vi "AB_1200_1100_Project_DestinationItems.vi"(6 "usedDestinations":i32[](array[numeric]), 7 "action":T2, 8 "error in (no error)":errorcluster, 9 "buildTypeGUID":string, 10 "oldBuildObject":T1, 11 "buildObject":T1) -> (0 "error out":errorcluster, 3 "buildObject out":T1)   [LabVIEW 2020]
doc: "Reads and writes the data to the object property bag."
uses:
  <resource>/Framework/Providers/API/ItemRef.ctl
  <vilib>/AppBuilder/RW_Project/AB_RW_Project_PropBag_ArrayAction.ctl
  <vilib>/AppBuilder/RW_Project/AB_RW_Project_PropBag_Action.ctl
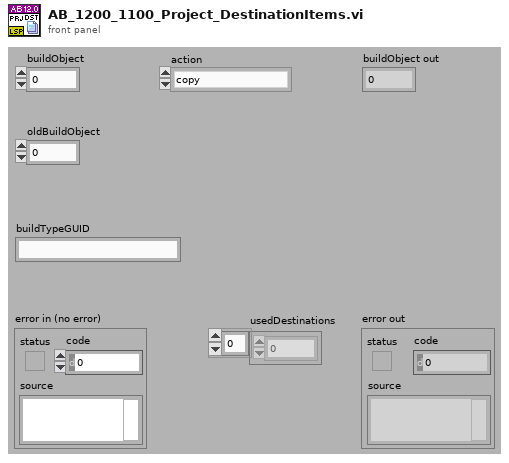
[diagram p1: front panel]
types:
  T1 = typedef "ItemRef.ctl" = u64
  T2 = typedef "AB_RW_Project_PropBag_ArrayAction.ctl" = enum16{"copy", "saveForPrevious", "loadFromPrevious", "clear"}
  T3 = typedef "AB_RW_Project_PropBag_Action.ctl" = enum16{"read", "write", "clear", "readPrevious", "writePrevious", "clearPrevious"}
  T4 = cluster{"destName":string, "path":path, "preserveHierarchy":bool, "libraryName":string}
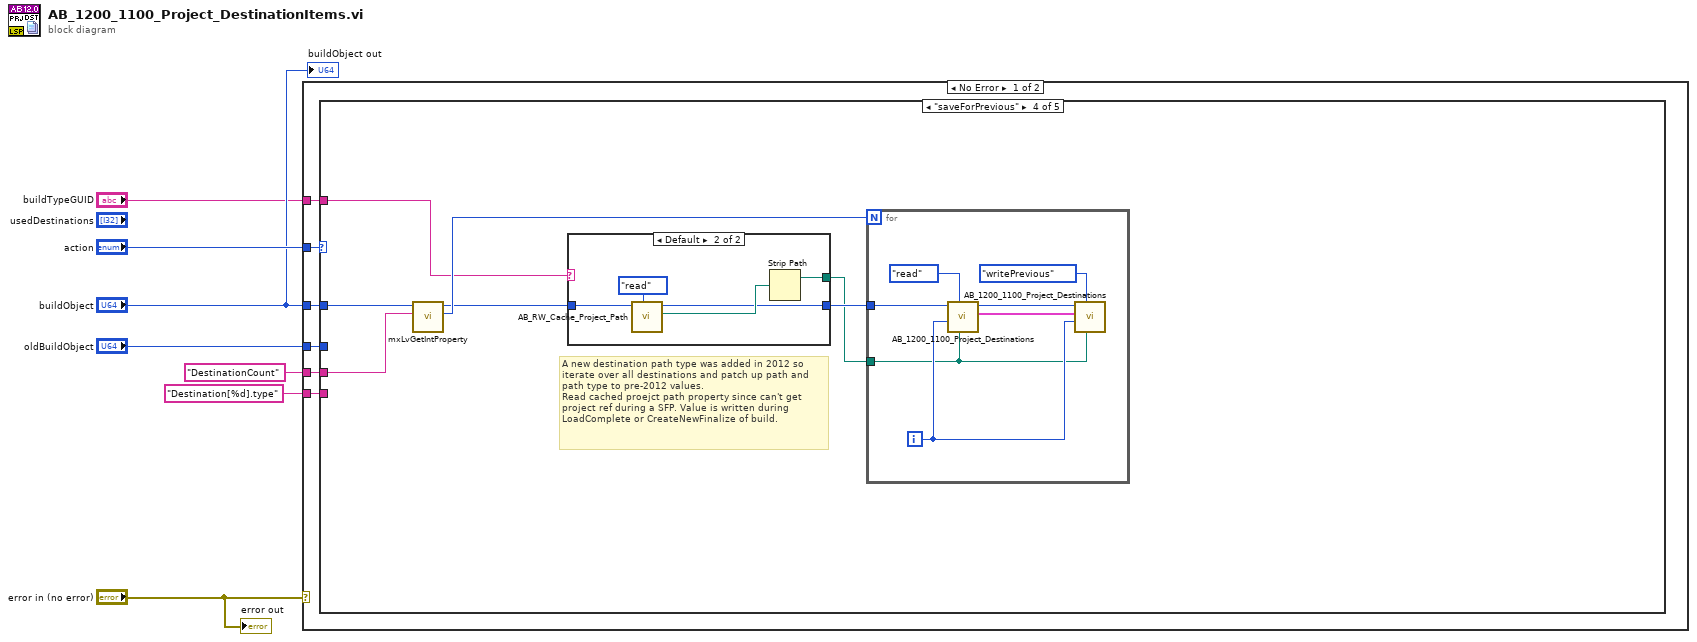
[diagram p0: block diagram]
diagram:
  n1 = case shown="No Error" "error in (no error)" {
    tunnel: "action" -> [w13 _]
    tunnel: "buildObject" -> [w12 _]
    tunnel: "DestinationCount" -> [w11 _]
    tunnel: "Destination[%d].type" -> [w10 _]
    tunnel: "oldBuildObject" -> [w9 _]
    tunnel: "buildTypeGUID" -> [w8 _]
    frame No Error {
      n2 = case shown="\"saveForPrevious\"" w13 {
        tunnel: w12 -> [_ _ _ w19 _]
        tunnel: w11 -> [_ _ _ w18 _]
        tunnel: w10 -> [_ _ _ _ _]
        tunnel: w9 -> [_ _ _ _ _]
        tunnel: w8 -> [_ _ _ w15 _]
        frame Default {
        }
        frame "loadFromPrevious" {
        }
        frame "copy" {
        }
        frame "saveForPrevious" {
          # "A new destination path type was added in 2012 so iterate over all destinations and patch up path and path type to pre-2012 values. \nRead cached proejct path property since can't get project ref during a SFP. Value is written during LoadComplete or CreateNewFinalize of build."
          n3 = call <resource>:"mxLvGetIntProperty.vi"("Tag"=w18, "Item"=w19) -> ("Value"=w20:i32, "Item"=w17:T1)  [unwired: 7 in, 1 out]
          n4 = case shown="Default" w15 {
            tunnel: w17 -> [w21 w23]
            tunnel: [w21 w22] -> w16
            tunnel: [_ w26] -> w14
            frame "{69A947D5-514E-4E75-818E-69657C0547D8}" {
              # "For RTEXE, destination items are saved as absolute"
            }
            frame Default {
              n5 = call <vilib>:"AB_RW_Cache_Project_Path.vi"("action"=AB_RW_Project_PropBag_Action."read", "buildObject"=w23) -> ("ProjectPath out"=w24:path, "buildObject out"=w22:T1)  [unwired: 7 in, 1 out]
              n6 = Strip Path(path=w24) -> (stripped path=w26:path)  [unwired: 1 out]
            }
          }
          n7 = for {
            N: w20 -> [_]
            tunnel: w16 -> [w32]
            tunnel: w14 -> [w28]
            i -> [w29]
            n8 = call <vilib>:"AB_1200_1100_Project_Destinations.vi"("ProjectPath"=w28, "action"=AB_RW_Project_PropBag_Action."read", "index"=w29, "buildObject"=w32) -> ("data out"=w27:T4, "buildObject out"=w31:T1)  [unwired: 4 in, 2 out]
            n9 = call <vilib>:"AB_1200_1100_Project_Destinations.vi"("ProjectPath"=w28, "action"=AB_RW_Project_PropBag_Action."writePrevious", "index"=w29, "data in"=w27, "buildObject"=w31) -> ()  [unwired: 3 in, 4 out]
          }
        }
        frame "clear" {
        }
      }
    }
    frame Error {
    }
  }
  "error out" <- "error in (no error)"
  "buildObject out" <- "buildObject"
